vi "Reference.vi"() -> ()   [LabVIEW 2020, in "Astemes_CSVReportPlugin.lvlib" / "Report Generator.lvlib"]
uses:
  Report Generator.lvlib
  Test Result Handler/TestStand Result Handler.lvclass
panel:
  in  "TestStand Result Handler":refnum<class "TestStand Result Handler.lvclass">
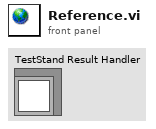
[diagram p1: front panel]
diagram:
